vi "Start Logic-Mode dependent case 2.vi"(6 "Case name string":string, 8 "error in (no error)":errorcluster, 9 "cancelled":bool, 10 "UI queue":refnum<queue>, 11 "Acq. queue in":refnum<queue>) -> (0 "error out":errorcluster, 3 "Acq. queue out":refnum<queue>)   [LabVIEW 2017]
uses:
  Queue/Message Queue/Typedefs/Message Cluster.ctl
  Typedefs/Read Write Enum.ctl
  Typedefs/Top level VI states.ctl
  Global Variables/gl_UI Ctrl Refs.vi
  Global Variables/General Globals.vi
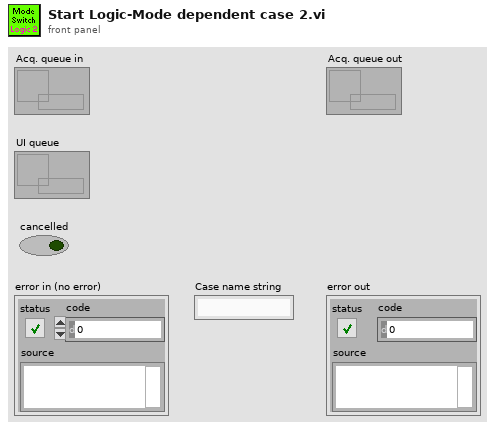
[diagram p1: front panel]
types:
  T1 = typedef "Read Write Enum.ctl" = enum16{"Read", "Write"}
  T2 = typedef "Top level VI states.ctl" = enum16{"None", "Initialise UI", "<STACK PROTOCOL STATES>", "AOL Zstack-START", "AOL Zstack-STOP", "Motor Zstack-START", "Motor Zstack-STOP", "<ACQUISITION PROTOCOL STATES> ", "Functional Acquisition-START", "Functional Acquisition-STOP", "Single Plane Acquisition-START", "Single Plane Acquisition-STOP", "Volume Acquisition-START", "Volume Acquisition-STOP", "<LIVE IMAGING PROTOCOL STATES>", "Live Imaging-START", "Live Imaging-STOP", "Live Plane Imaging-START", "Live Plane Imaging-STOP", "Live Volume Imaging-START", "Live Volume Imaging-STOP", "<MOVEMENT CORRECTION PROTOCOL STATES>", "EXIT"}
  T3 = typedef "UI ctrl refs cluster.ctl" = cluster{"Top level VI path":path, "Top level VI ref":refnum<vi>, "User menu ref":refnum<k9>, "Sub Panel control":refnum<vi>, "Imaging Param Tab":refnum<vi>, "Occurrence-Start drivers":refnum<k4>, "Occurrence-Speed logging initialised":refnum<k4>, "Occurrence-XYZ stage initialised":refnum<k4>, "Exit button":refnum<vi>, "Status ind":refnum<vi>, "Set as origin":refnum<vi>, "Speed Logging":refnum<vi>, "Time Lapse":refnum<vi>, "Live Imaging":refnum<vi>, "AOL Z Stack":refnum<vi>, "Motor Z Stack":refnum<vi>, "Funct Acq button":refnum<vi>, "Hard Shutter":refnum<vi>, "Virtual Shutter":refnum<vi>, "Laser Power":refnum<vi>, "AOL Mode":refnum<vi>, "Frame Size":refnum<vi>, "Field of View":refnum<vi>, "Dwell Time":refnum<vi>, "Zoom":refnum<vi>, "AOL Z":refnum<vi>, "Objective":refnum<vi>, "Axis":refnum<vi>, "Paths & Names":refnum<vi>, "Experiment folder path (ind.)":refnum<vi>, "Last State (Ind.)":refnum<vi>, "Averages":refnum<vi>, "Angle (degrees)":refnum<vi>, "X centre":refnum<vi>, "Y centre":refnum<vi>, "Plane Mode":refnum<vi>, "# Planes":refnum<vi>, "Z Start":refnum<vi>, "Z Stop":refnum<vi>, "Z Step":refnum<vi>, "PMT 1":refnum<vi>, "PMT 2":refnum<vi>, "Stage XYZ Position":refnum<vi>, "Pockels@Z Start":refnum<vi>, "Pockels@Z Stop":refnum<vi>, "Obtain Z Start":refnum<vi>, "Obtain Z Stop":refnum<vi>, "Live stim.trig.period":refnum<vi>, "Live stim.trig.enable":refnum<vi>, "Movement Correction":refnum<vi>, "Load Reference Image":refnum<vi>, "XY Stage Move":refnum<vi>, "MovCor Cluster":refnum<vi>, "RefDAQParam":refnum<vi>, "Funct. Acq. Pockels Modulation":refnum<vi>, "Ref Laser Power":refnum<vi>, "Enable Video Recording":refnum<vi>, "Video Record-Live Imaging":refnum<vi>, "Video Record-Funct acq":refnum<vi>, "Reference Source":refnum<vi>, "AOL Z-stack Chirps Ready (ind)":refnum<vi>, "Target time between mov.cor. ref triggers (ms)":refnum<vi>, "Funct. Acq. Ref frame save":refnum<vi>, "Tracking button":refnum<vi>, "Show ref plots window":refnum<vi>, "Center freq ind (nm)":refnum<vi>, "Pickup mode (ind)":refnum<vi>, "Logging queue (ind)":refnum<vi>, "Back aperture power (ind.)":refnum<vi>, "Power after objective (ind.)":refnum<vi>, "Switch user":refnum<vi>, "Ls1 Conn. Status":refnum<vi>, "Ls1Tuning Status":refnum<vi>, "Ls1 Faults":refnum<vi>, "Ls1 Connection":refnum<vi>, "Ls1 Mode":refnum<vi>, "Ls1 POWER [mW]":refnum<vi>, "Ls1Shutter":refnum<vi>, "Ls1 Wavelength":refnum<vi>, "Ls1 Note":refnum<vi>, "Ls1 Confirm Wav":refnum<vi>, "Ls1 PreChrp Prism1":refnum<vi>, "Ls1 PreChrp Prism2":refnum<vi>, "Ls1 wav top Ind":refnum<vi>, "Ls1 power top Ind":refnum<vi>, "Ls1 Pump peak Hold":refnum<vi>, "Ls1 Status Ind":refnum<vi>, "Ls1 wav cancel":refnum<vi>, "Experiment Type":refnum<vi>, "Biology Information":refnum<vi>}
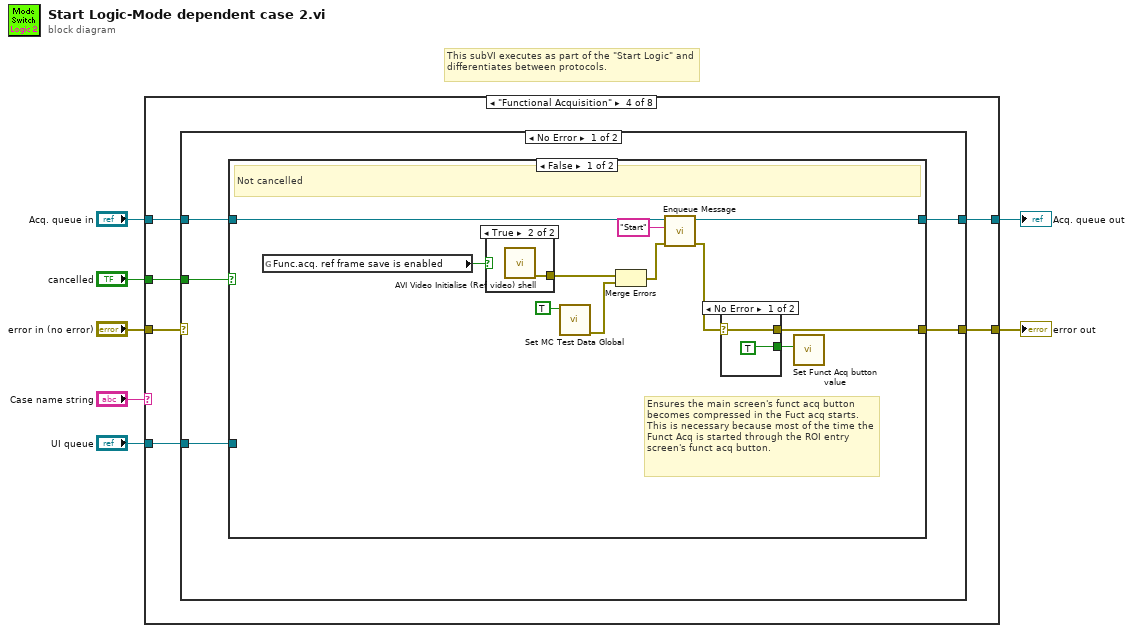
[diagram p0: block diagram]
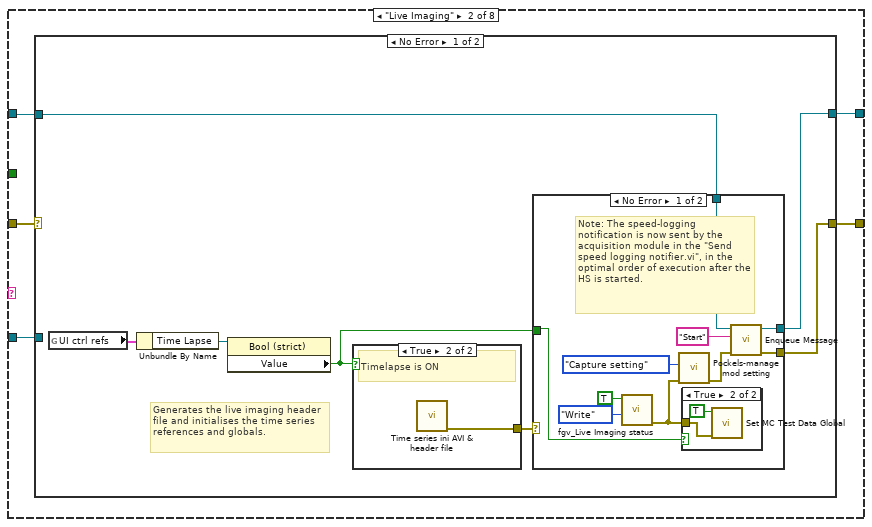
[diagram p3: hidden frame]
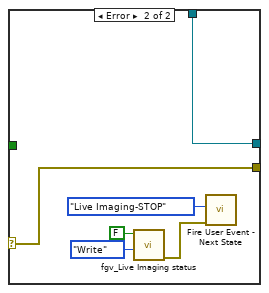
[diagram p5: hidden frame]
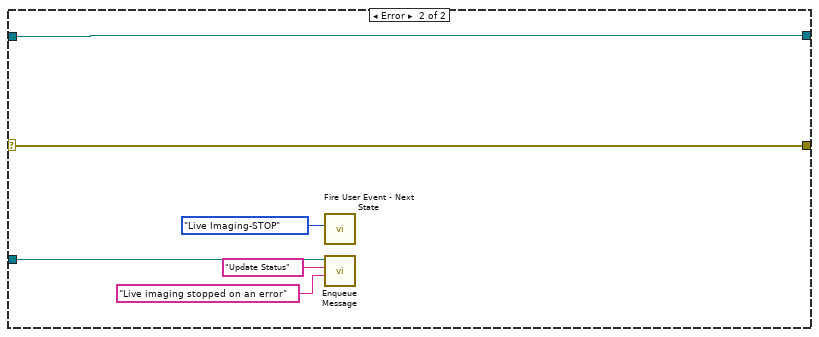
[diagram p7: hidden frame]
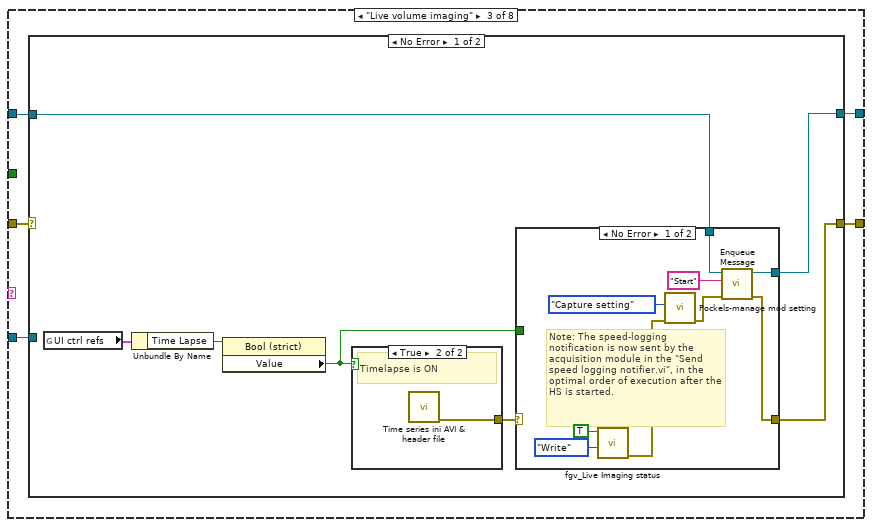
[diagram p8: hidden frame]
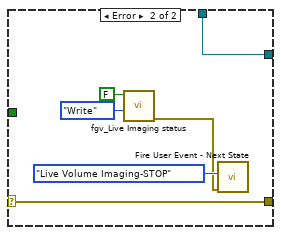
[diagram p9: hidden frame]
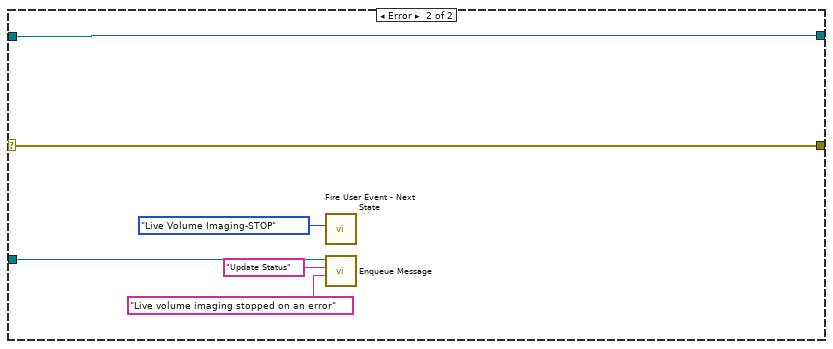
[diagram p11: hidden frame]
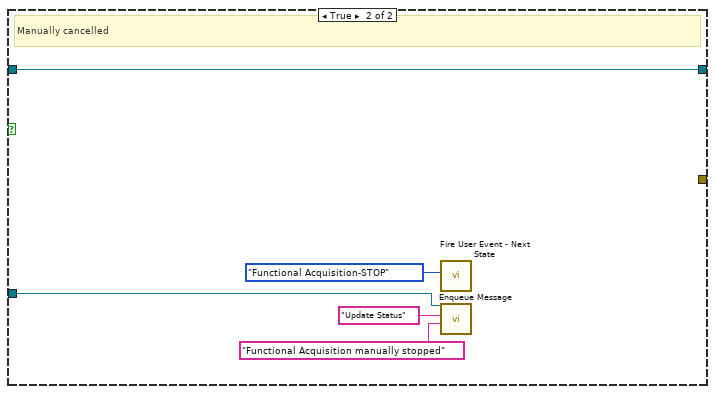
[diagram p14: hidden frame]
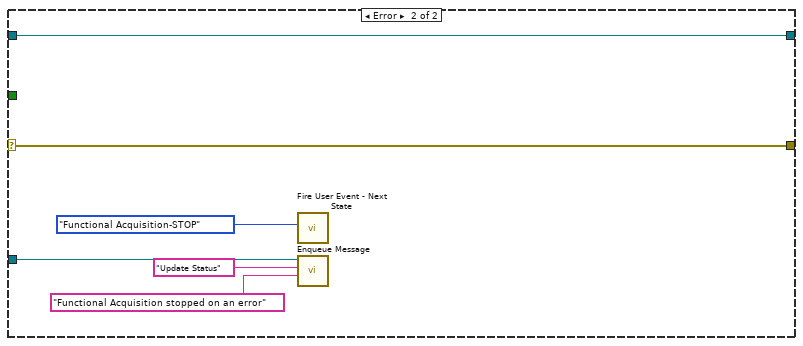
[diagram p15: hidden frame]
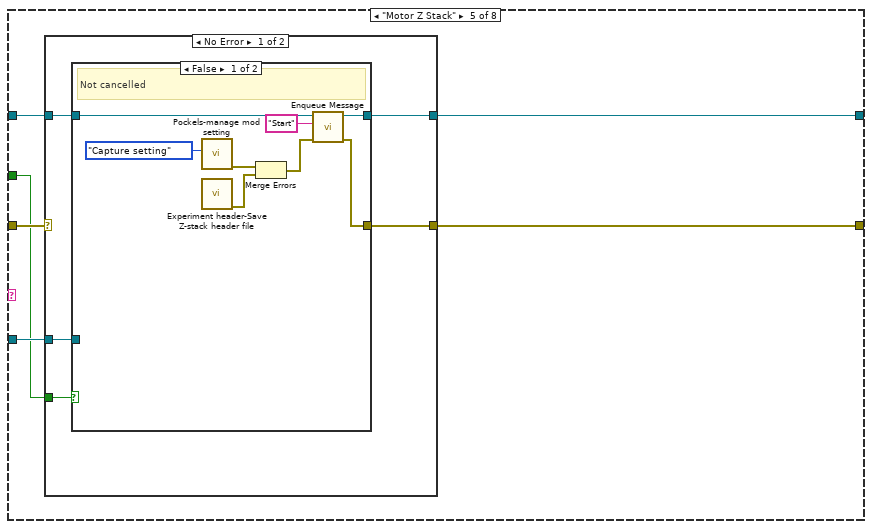
[diagram p16: hidden frame]
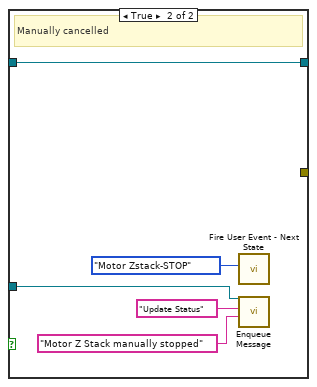
[diagram p17: hidden frame]
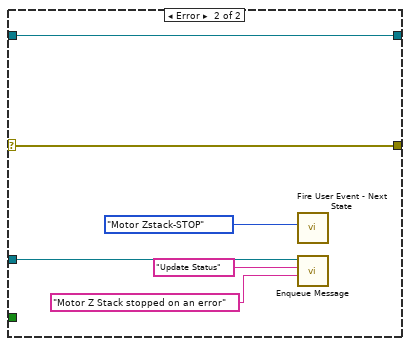
[diagram p18: hidden frame]
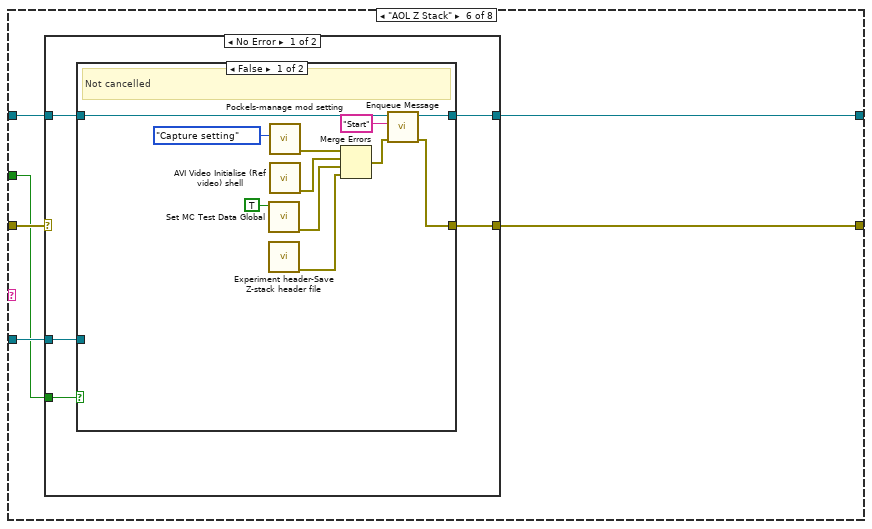
[diagram p19: hidden frame]
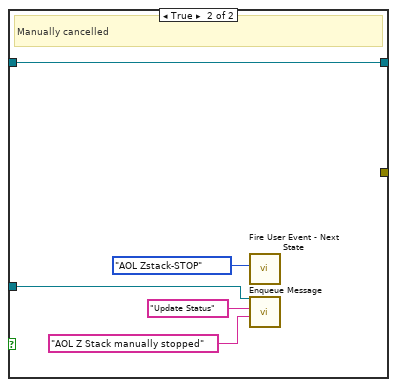
[diagram p20: hidden frame]
diagram:
  # "This subVI executes as part of the \"Start Logic\" and differentiates between protocols."
  n1 = case shown="\"Functional Acquisition\"" "Case name string" {
    tunnel: [w9 w14 w51 w83 w120 w150 w183 w213] -> w1
    tunnel: "error in (no error)" -> [w9 w11 w48 w84 w121 w151 w184 w214]
    tunnel: [w8 w12 w49 w86 w123 w153 w186 w216] -> w3
    tunnel: "Acq. queue in" -> [w8 w13 w50 w85 w122 w152 w185 w215]
    tunnel: "UI queue" -> [_ w10 w47 w82 w119 w149 w182 w212]
    tunnel: "cancelled" -> [_ _ _ w81 w118 w148 w181 w211]
    frame Default {
    }
    frame "Live Imaging" {
      n2 = case shown="No Error" w11 {
        selector: w11 -> [_ w46]
        tunnel: [w16 w46] -> w14
        tunnel: w13 -> [w18 w45]
        tunnel: [w17 w45] -> w12
        tunnel: w10 -> [_ w41]
        frame No Error {
          # "Generates the live imaging header file and initialises the time series references and globals."
          n3 = global read "gl_UI Ctrl Refs.vi" "UI ctrl refs"() -> (w15:T3)
          n4 = Unbundle By Name(w15) -> ("Time Lapse"=w21:refnum<vi>)
          n5 = property class="Bool (strict)"(reference=w21) -> ("Value"=w19:bool)  [unwired: 1 in, 2 out]
          n6 = case shown="True" w19 {
            tunnel: [_ w40] -> w20
            frame False {
              # "Timelapse is OFF"
            }
            frame True {
              # "Timelapse is ON"
              n7 = call "Time series ini AVI & header file.vi"() -> ("error out"=w40:errorcluster)  [unwired: 11 in]
            }
          }
          n8 = case shown="No Error" w20 {
            selector: w20 -> [_ w37]
            tunnel: w19 -> [w22 _]
            tunnel: w18 -> [w28 w38]
            tunnel: [w30 w38] -> w17
            tunnel: [w29 w37] -> w16
            frame No Error {
              # "Note: The speed-logging notification is now sent by the acquisition module in the \"Send speed logging notifier.vi\", in the optimal order of execution after the HS is started."
              n9 = call "fgv_Live Imaging status.vi"("Function"=Read_Write_Enum."Write", "Live Imaging?"=TRUE ("Timelapse?")) -> ("error out"=w23:errorcluster)  [unwired: 8 in, 1 out]
              n10 = call "Pockels-manage mod setting.vi"("error in (no error)"=w23, "Function"=enum16{"Capture setting", "Re-apply setting"}."Capture setting") -> ("error out"=w27:errorcluster)  [unwired: 9 in]
              n11 = case shown="True" w22 {
                tunnel: w23 -> [_ w32]
                frame False {
                }
                frame True {
                  n12 = call "Set MC Test Data Global.vi"("error in (no error)"=w32, "Save MC TestData"=TRUE) -> ()  [unwired: 9 in, 1 out]
                }
              }
              n13 = call "Enqueue Message.vi"("error in (no error)"=w27, "Message"="Start", "Queue"=w28) -> ("error out"=w29:errorcluster, "Queue out"=w30:refnum<queue>)  [unwired: 7 in]
            }
            frame Error {
              n14 = call "fgv_Live Imaging status.vi"("Function"=Read_Write_Enum."Write", "Live Imaging?"=FALSE ("Timelapse?")) -> ("error out"=w34:errorcluster)  [unwired: 8 in, 1 out]
              n15 = call "Fire User Event - Next State.vi"("Error In"=w34, "\"UI Handler loop\" case to execute"=Top_level_VI_states."Live Imaging-STOP" ("event data / imaging mode")) -> ()  [unwired: 9 in, 1 out]
            }
          }
        }
        frame Error {
          n16 = call "Fire User Event - Next State.vi"("\"UI Handler loop\" case to execute"=Top_level_VI_states."Live Imaging-STOP" ("event data / imaging mode")) -> ()  [unwired: 10 in, 1 out]
          n17 = call "Enqueue Message.vi"("Message Data"="Live imaging stopped on an error" ("Acquiring and Logging..."), "Message"="Update Status", "Queue"=w41) -> ()  [unwired: 7 in, 2 out]
        }
      }
    }
    frame "Live volume imaging" {
      n18 = case shown="No Error" w48 {
        selector: w48 -> [_ w80]
        tunnel: [w55 w80] -> w51
        tunnel: w50 -> [w54 w79]
        tunnel: [w53 w79] -> w49
        tunnel: w47 -> [_ w76]
        frame No Error {
          n19 = global read "gl_UI Ctrl Refs.vi" "UI ctrl refs"() -> (w52:T3)
          n20 = Unbundle By Name(w52) -> ("Time Lapse"=w58:refnum<vi>)
          n21 = property class="Bool (strict)"(reference=w58) -> ("Value"=w56:bool)  [unwired: 1 in, 2 out]
          n22 = case shown="True" w56 {
            tunnel: [_ w74] -> w57
            frame False {
              # "Timelapse is OFF"
            }
            frame True {
              # "Timelapse is ON"
              n23 = call "Time series ini AVI & header file.vi"() -> ("error out"=w74:errorcluster)  [unwired: 11 in]
            }
          }
          n24 = case shown="No Error" w57 {
            selector: w57 -> [_ w73]
            tunnel: [w66 w73] -> w55
            tunnel: w56 -> [_ _]
            tunnel: w54 -> [w65 w71]
            tunnel: [w64 w71] -> w53
            frame No Error {
              # "Note: The speed-logging notification is now sent by the acquisition module in the \"Send speed logging notifier.vi\", in the optimal order of execution after the HS is started."
              n25 = call "fgv_Live Imaging status.vi"("Function"=Read_Write_Enum."Write", "Live Imaging?"=TRUE ("Timelapse?")) -> ("error out"=w59:errorcluster)  [unwired: 8 in, 1 out]
              n26 = call "Pockels-manage mod setting.vi"("error in (no error)"=w59, "Function"=enum16{"Capture setting", "Re-apply setting"}."Capture setting") -> ("error out"=w63:errorcluster)  [unwired: 9 in]
              n27 = call "Enqueue Message.vi"("error in (no error)"=w63, "Message"="Start", "Queue"=w65) -> ("error out"=w66:errorcluster, "Queue out"=w64:refnum<queue>)  [unwired: 7 in]
            }
            frame Error {
              n28 = call "fgv_Live Imaging status.vi"("Function"=Read_Write_Enum."Write", "Live Imaging?"=FALSE ("Timelapse?")) -> ("error out"=w68:errorcluster)  [unwired: 8 in, 1 out]
              n29 = call "Fire User Event - Next State.vi"("Error In"=w68, "\"UI Handler loop\" case to execute"=Top_level_VI_states."Live Volume Imaging-STOP" ("event data / imaging mode")) -> ()  [unwired: 9 in, 1 out]
            }
          }
        }
        frame Error {
          n30 = call "Fire User Event - Next State.vi"("\"UI Handler loop\" case to execute"=Top_level_VI_states."Live Volume Imaging-STOP" ("event data / imaging mode")) -> ()  [unwired: 10 in, 1 out]
          n31 = call "Enqueue Message.vi"("Message Data"="Live volume imaging stopped on an error" ("Acquiring and Logging..."), "Message"="Update Status", "Queue"=w76) -> ()  [unwired: 7 in, 2 out]
        }
      }
    }
    frame "Functional Acquisition" {
      n32 = case shown="No Error" w84 {
        selector: w84 -> [_ w116]
        tunnel: [w87 w116] -> w83
        tunnel: [w88 w117] -> w86
        tunnel: w85 -> [w89 w117]
        tunnel: w82 -> [w91 w112]
        tunnel: w81 -> [w90 _]
        frame No Error {
          n33 = case shown="False" w90 {
            tunnel: w91 -> [_ w108]
            tunnel: w89 -> [w101 w107]
            tunnel: [w100 w107] -> w88
            tunnel: [w94 _] -> w87
            frame False {
              # "Ensures the main screen's funct acq button becomes compressed in the Fuct acq starts. This is necessary because most of the time the Funct Acq is started through the ROI entry screen's funct acq button."
              # "Not cancelled"
              n34 = global read "General Globals.vi" "Func.acq. ref frame save is enabled"() -> (w96:bool)
              n35 = case shown="True" w96 {
                tunnel: [_ w106] -> w92
                frame False {
                }
                frame True {
                  n36 = call "AVI Video Initialise (Ref video) shell.vi"() -> ("error out"=w106:errorcluster)  [unwired: 11 in]
                }
              }
              n37 = call "Set MC Test Data Global.vi"("Save MC TestData"=TRUE) -> ("error out"=w98:errorcluster)  [unwired: 10 in]
              n38 = Merge Errors(w92, w98) -> (w97:errorcluster)
              n39 = call "Enqueue Message.vi"("error in (no error)"=w97, "Message"="Start", "Queue"=w101) -> ("error out"=w95:errorcluster, "Queue out"=w100:refnum<queue>)  [unwired: 7 in]
              n40 = case shown="No Error" w95 {
                selector: w95 -> [w104 w105]
                tunnel: [w104 w105] -> w94
                tunnel: [TRUE ("Value") _] -> w93
                frame No Error {
                }
                frame Error {
                }
              }
              n41 = call "Set Funct Acq button value.vi"("Functional Acquisition button's new value"=w93) -> ()  [unwired: 10 in, 1 out]
            }
            frame True {
              # "Manually cancelled"
              n42 = call "Fire User Event - Next State.vi"("\"UI Handler loop\" case to execute"=Top_level_VI_states."Functional Acquisition-STOP" ("event data / imaging mode")) -> ()  [unwired: 10 in, 1 out]
              n43 = call "Enqueue Message.vi"("Message Data"="Functional Acquisition manually stopped" ("Acquiring and Logging..."), "Message"="Update Status", "Queue"=w108) -> ()  [unwired: 7 in, 2 out]
            }
          }
        }
        frame Error {
          n44 = call "Fire User Event - Next State.vi"("\"UI Handler loop\" case to execute"=Top_level_VI_states."Functional Acquisition-STOP" ("event data / imaging mode")) -> ()  [unwired: 10 in, 1 out]
          n45 = call "Enqueue Message.vi"("Message Data"="Functional Acquisition stopped on an error" ("Acquiring and Logging..."), "Message"="Update Status", "Queue"=w112) -> ()  [unwired: 7 in, 2 out]
        }
      }
    }
    frame "Motor Z Stack" {
      n46 = case shown="No Error" w121 {
        selector: w121 -> [_ w146]
        tunnel: [w124 w146] -> w120
        tunnel: [w125 w147] -> w123
        tunnel: w122 -> [w126 w147]
        tunnel: w119 -> [w128 w142]
        tunnel: w118 -> [w127 _]
        frame No Error {
          n47 = case shown="False" w127 {
            tunnel: w128 -> [_ w138]
            tunnel: w126 -> [w135 w137]
            tunnel: [w134 w137] -> w125
            tunnel: [w133 _] -> w124
            frame False {
              # "Not cancelled"
              n48 = call "Pockels-manage mod setting.vi"("Function"=enum16{"Capture setting", "Re-apply setting"}."Capture setting") -> ("error out"=w131:errorcluster)  [unwired: 10 in]
              n49 = call "Experiment header-Save Z-stack header file.vi"() -> ("error out"=w130:errorcluster)  [unwired: 11 in]
              n50 = Merge Errors(w131, w130) -> (w129:errorcluster)
              n51 = call "Enqueue Message.vi"("error in (no error)"=w129, "Message"="Start", "Queue"=w135) -> ("error out"=w133:errorcluster, "Queue out"=w134:refnum<queue>)  [unwired: 7 in]
            }
            frame True {
              # "Manually cancelled"
              n52 = call "Fire User Event - Next State.vi"("\"UI Handler loop\" case to execute"=Top_level_VI_states."Motor Zstack-STOP" ("event data / imaging mode")) -> ()  [unwired: 10 in, 1 out]
              n53 = call "Enqueue Message.vi"("Message Data"="Motor Z Stack manually stopped" ("Acquiring and Logging..."), "Message"="Update Status", "Queue"=w138) -> ()  [unwired: 7 in, 2 out]
            }
          }
        }
        frame Error {
          n54 = call "Fire User Event - Next State.vi"("\"UI Handler loop\" case to execute"=Top_level_VI_states."Motor Zstack-STOP" ("event data / imaging mode")) -> ()  [unwired: 10 in, 1 out]
          n55 = call "Enqueue Message.vi"("Message Data"="Motor Z Stack stopped on an error" ("Acquiring and Logging..."), "Message"="Update Status", "Queue"=w142) -> ()  [unwired: 7 in, 2 out]
        }
      }
    }
    frame "AOL Z Stack" {
      n56 = case shown="No Error" w151 {
        selector: w151 -> [_ w179]
        tunnel: [w154 w179] -> w150
        tunnel: [w155 w180] -> w153
        tunnel: w152 -> [w156 w180]
        tunnel: w149 -> [w158 w175]
        tunnel: w148 -> [w157 _]
        frame No Error {
          n57 = case shown="False" w157 {
            tunnel: w158 -> [_ w171]
            tunnel: w156 -> [w168 w170]
            tunnel: [w167 w170] -> w155
            tunnel: [w166 _] -> w154
            frame False {
              # "Not cancelled"
              n58 = call "Set MC Test Data Global.vi"("Save MC TestData"=TRUE) -> ("error out"=w160:errorcluster)  [unwired: 10 in]
              n59 = call "Experiment header-Save Z-stack header file.vi"() -> ("error out"=w159:errorcluster)  [unwired: 11 in]
              n60 = call "Pockels-manage mod setting.vi"("Function"=enum16{"Capture setting", "Re-apply setting"}."Capture setting") -> ("error out"=w164:errorcluster)  [unwired: 10 in]
              n61 = call "AVI Video Initialise (Ref video) shell.vi"() -> ("error out"=w162:errorcluster)  [unwired: 11 in]
              n62 = Merge Errors(w164, w162, w160, w159) -> (w163:errorcluster)
              n63 = call "Enqueue Message.vi"("error in (no error)"=w163, "Message"="Start", "Queue"=w168) -> ("error out"=w166:errorcluster, "Queue out"=w167:refnum<queue>)  [unwired: 7 in]
            }
            frame True {
              # "Manually cancelled"
              n64 = call "Fire User Event - Next State.vi"("\"UI Handler loop\" case to execute"=Top_level_VI_states."AOL Zstack-STOP" ("event data / imaging mode")) -> ()  [unwired: 10 in, 1 out]
              n65 = call "Enqueue Message.vi"("Message Data"="AOL Z Stack manually stopped" ("Acquiring and Logging..."), "Message"="Update Status", "Queue"=w171) -> ()  [unwired: 7 in, 2 out]
            }
          }
        }
        frame Error {
          n66 = call "Fire User Event - Next State.vi"("\"UI Handler loop\" case to execute"=Top_level_VI_states."AOL Zstack-STOP" ("event data / imaging mode")) -> ()  [unwired: 10 in, 1 out]
          n67 = call "Enqueue Message.vi"("Message Data"="AOL Z Stack stopped on an error" ("Acquiring and Logging..."), "Message"="Update Status", "Queue"=w175) -> ()  [unwired: 7 in, 2 out]
        }
      }
    }
    frame "Volume acquisition" {
      n68 = case shown="No Error" w184 {
        selector: w184 -> [_ w209]
        tunnel: [w187 w209] -> w183
        tunnel: [w188 w210] -> w186
        tunnel: w185 -> [w189 w210]
        tunnel: w182 -> [w191 w205]
        tunnel: w181 -> [w190 _]
        frame No Error {
          n69 = case shown="False" w190 {
            tunnel: w191 -> [_ w201]
            tunnel: w189 -> [w198 w200]
            tunnel: [w197 w200] -> w188
            tunnel: [w196 _] -> w187
            frame False {
              # "Not cancelled"
              n70 = call "AVI Video Initialise (Ref video) shell.vi"() -> ("error out"=w193:errorcluster)  [unwired: 11 in]
              n71 = call "Set MC Test Data Global.vi"("Save MC TestData"=TRUE) -> ("error out"=w194:errorcluster)  [unwired: 10 in]
              n72 = Merge Errors(w193, w194) -> (w192:errorcluster)
              n73 = call "Enqueue Message.vi"("error in (no error)"=w192, "Message"="Start", "Queue"=w198) -> ("error out"=w196:errorcluster, "Queue out"=w197:refnum<queue>)  [unwired: 7 in]
            }
            frame True {
              # "Manually cancelled"
              n74 = call "Fire User Event - Next State.vi"("\"UI Handler loop\" case to execute"=Top_level_VI_states."Volume Acquisition-STOP" ("event data / imaging mode")) -> ()  [unwired: 10 in, 1 out]
              n75 = call "Enqueue Message.vi"("Message Data"="Volume Acquisition manually stopped" ("Acquiring and Logging..."), "Message"="Update Status", "Queue"=w201) -> ()  [unwired: 7 in, 2 out]
            }
          }
        }
        frame Error {
          n76 = call "Fire User Event - Next State.vi"("\"UI Handler loop\" case to execute"=Top_level_VI_states."Volume Acquisition-STOP" ("event data / imaging mode")) -> ()  [unwired: 10 in, 1 out]
          n77 = call "Enqueue Message.vi"("Message Data"="Volume Acquisition stopped on an error" ("Acquiring and Logging..."), "Message"="Update Status", "Queue"=w205) -> ()  [unwired: 7 in, 2 out]
        }
      }
    }
    frame "Single Plane Acquisition" {
      n78 = case shown="No Error" w214 {
        selector: w214 -> [_ w239]
        tunnel: [w217 w239] -> w213
        tunnel: [w218 w240] -> w216
        tunnel: w215 -> [w219 w240]
        tunnel: w212 -> [w221 w235]
        tunnel: w211 -> [w220 _]
        frame No Error {
          n79 = case shown="True" w220 {
            tunnel: w221 -> [_ w231]
            tunnel: w219 -> [w228 w230]
            tunnel: [w227 w230] -> w218
            tunnel: [w226 _] -> w217
            frame False {
              # "Not cancelled"
              n80 = call "Pockels-manage mod setting.vi"("Function"=enum16{"Capture setting", "Re-apply setting"}."Capture setting") -> ("error out"=w224:errorcluster)  [unwired: 10 in]
              n81 = call "AVI Video Initialise (Ref video) shell.vi"() -> ("error out"=w223:errorcluster)  [unwired: 11 in]
              n82 = Merge Errors(w224, w223) -> (w222:errorcluster)
              n83 = call "Enqueue Message.vi"("error in (no error)"=w222, "Message"="Start", "Queue"=w228) -> ("error out"=w226:errorcluster, "Queue out"=w227:refnum<queue>)  [unwired: 7 in]
            }
            frame True {
              # "Manually cancelled"
              n84 = call "Fire User Event - Next State.vi"("\"UI Handler loop\" case to execute"=Top_level_VI_states."Single Plane Acquisition-STOP" ("event data / imaging mode")) -> ()  [unwired: 10 in, 1 out]
              n85 = call "Enqueue Message.vi"("Message Data"="Single Plane Acquisition manually stopped" ("Acquiring and Logging..."), "Message"="Update Status", "Queue"=w231) -> ()  [unwired: 7 in, 2 out]
            }
          }
        }
        frame Error {
          n86 = call "Fire User Event - Next State.vi"("\"UI Handler loop\" case to execute"=Top_level_VI_states."Single Plane Acquisition-STOP" ("event data / imaging mode")) -> ()  [unwired: 10 in, 1 out]
          n87 = call "Enqueue Message.vi"("Message Data"="Single Plane Acquisition stopped on an error" ("Acquiring and Logging..."), "Message"="Update Status", "Queue"=w235) -> ()  [unwired: 7 in, 2 out]
        }
      }
    }
  }
  "Acq. queue out" <- w3
  "error out" <- w1
